vi "LV8_8.vi"() -> ()   [LabVIEW 2016]
uses:
  <vilib>/sound2/lvsound2.llb/Sampling Mode.ctl
  <vilib>/Utility/file.llb/Read From Spreadsheet File (DBL).vi
  <vilib>/imath/engines/lvmath2/RunTimeEngine/BuiltInFunctions/length/NIMS_length(GV).vi
  <instcachedir>/0/NIMS_length(GV)_08A3D13377FD4E4B96F5795FBF3698FA.lvgen/NIMS_length(GV)_08A3D13377FD4E4B96F5795FBF3698FA_000.vi
  <vilib>/imath/engines/lvmath2/RunTimeEngine/BuiltInFunctions/fft/NIMS_fft(GV).vi
  <instcachedir>/0/NIMS_fft(GV)_4C6467FC22F84E4BA42517A07EF978B0.lvgen/NIMS_fft(GV)_4C6467FC22F84E4BA42517A07EF978B0_000.vi
  <vilib>/imath/engines/lvmath2/RunTimeEngine/ErrorHandling/NIMS_Error From Error Code.vi
  <vilib>/imath/engines/lvmath2/RunTimeEngine/BuiltInFunctions/round/NIMS_round(DBL-S).vi
  <vilib>/imath/engines/lvmath2/RunTimeEngine/RangeToken/NIMS_Range_R2 - Integer.vi
  <instcachedir>/0/NIMS_Range_R2 - Integer_89B873E74E6E489885E44F751DD9C6BF.lvgen/NIMS_Range_R2 - Integer_89B873E74E6E489885E44F751DD9C6BF_000.vi
  <vilib>/imath/engines/lvmath2/RunTimeEngine/CommandStatement/MC_CommandStatement_break.vi
  <vilib>/imath/engines/lvmath2/RunTimeEngine/RowToken/NIMS_RowToken_M_SorRV.vi
  <instcachedir>/0/NIMS_RowToken_M_SorRV_4D710C5E6F8040F3A39B2F03436798DB.lvgen/NIMS_RowToken_M_SorRV_4D710C5E6F8040F3A39B2F03436798DB_000.vi
  <vilib>/imathl/engines/lvmath/Functions/Error Handling/Create Error.vi
  <vilib>/imath/engines/lvmath2/RunTimeEngine/RowToken/NIMS_RowToken_M_M.vi
  <instcachedir>/0/NIMS_RowToken_M_M_968CDE3545E74ACDAEA4B48DE01EEECA.lvgen/NIMS_RowToken_M_M_968CDE3545E74ACDAEA4B48DE01EEECA_004.vi
  <vilib>/imath/engines/lvmath2/RunTimeEngine/IndexReplace/NIMS V(M)=S.vi
  <instcachedir>/0/NIMS V(M)=S_9709F0D32A8A4ECDA1CDD54D8B4B61B5.lvgen/NIMS V(M)=S_9709F0D32A8A4ECDA1CDD54D8B4B61B5_000.vi
  <vilib>/imath/engines/lvmath2/RunTimeSupport/NIMS_Error if Not Equal.vi
  <instcachedir>/0/NIMS_Error if Not Equal_43252A79AD05436189442EC0C5E5AB8A.lvgen/NIMS_Error if Not Equal_43252A79AD05436189442EC0C5E5AB8A_002.vi
  <vilib>/imath/engines/lvmath2/RunTimeEngine/ErrorHandling/NIMS_Create Error From Enums.vi
  <vilib>/imath/engines/lvmath2/RunTimeEngine/BuiltInFunctions/ifft/NIMS_ifft(CV).vi
  <vilib>/imath/engines/lvmath2/RunTimeEngine/IndexRead/NIMS V(V).vi
  <instcachedir>/0/NIMS V(V)_298D9CB7BFEB42B8BC8D9C3C28AE8C70.lvgen/NIMS V(V)_298D9CB7BFEB42B8BC8D9C3C28AE8C70_000.vi
  <vilib>/imath/engines/lvmath2/RunTimeEngine/BuiltInFunctions/abs/NIMS_abs(signed).vi
  <instcachedir>/0/NIMS_abs(signed)_C4FCB8E6058B49B797C7C8D53CA5F6EC.lvgen/NIMS_abs(signed)_C4FCB8E6058B49B797C7C8D53CA5F6EC_006.vi
  <vilib>/imath/engines/lvmath2/RunTimeEngine/NodeEndStatement/NIMS_NodeEndStatement_Output.vi
  <instcachedir>/0/NIMS_NodeEndStatement_Output_53EC0D466D134D7ABD903AC30B43404B.lvgen/NIMS_NodeEndStatement_Output_53EC0D466D134D7ABD903AC30B43404B_005.vi
  <instcachedir>/0/NIMS_NodeEndStatement_Output_53EC0D466D134D7ABD903AC30B43404B.lvgen/NIMS_NodeEndStatement_Output_53EC0D466D134D7ABD903AC30B43404B_010.vi
  <vilib>/imath/engines/lvmath2/RunTimeEngine/ErrorHandling/NIMS_Finalize Error.vi
  <vilib>/sound2/lvsound2.llb/Sound Output Write (DBL Single).vi
panel:
  out "?":dbl
  in  "Fundamental rejection frequency":dbl(slide)=436.0 scale=400.0..500.0
  out "Filtered (frequency domain)":cluster{"F":dbl[], "FYI":dbl[]}(graph)
  out "Original signal (frequency domain)":cluster{"F":dbl[], "FXI":dbl[]}(graph)
  out "Original signal (time domain)":cluster{"t":dbl[], "first row":dbl[]}(graph)={"t"=[0.022675736961451247, 0.022698412698412697, 0.02272108843537415, 0.0227437641723356, 0.022766439909297054, 0.022789115646258504, 0.022811791383219954, 0.022834467120181407, 0.022857142857142857, 0.022879818594104307, 0.02290249433106576, 0.02292517006802721, 0.02294784580498866, 0.022970521541950114, 0.022993197278911564, 0.023015873015873017, 0.023038548752834467, 0.023061224489795917, 0.02308390022675737, 0.02310657596371882, 0.02312925170068027, 0.023151927437641724, 0.023174603174603174, 0.023197278911564624, 0.023219954648526078, 0.023242630385487528, 0.02326530612244898, 0.02328798185941043, 0.02331065759637188, 0.023333333333333334, 0.023356009070294784, 0.023378684807256234, 0.023401360544217688, 0.023424036281179138, 0.02344671201814059, 0.02346938775510204, 0.02349206349206349, 0.023514739229024945, 0.023537414965986395, 0.023560090702947845, 0.023582766439909298, 0.023605442176870748, 0.023628117913832198, 0.02365079365079365, 0.0236734693877551, 0.023696145124716555, 0.023718820861678005, 0.023741496598639455, 0.023764172335600908, 0.023786848072562358, 0.023809523809523808, 0.02383219954648526, 0.02385487528344671, 0.02387755102040816, 0.023900226757369615, 0.023922902494331065, 0.02394557823129252, 0.02396825396825397, 0.02399092970521542, 0.024013605442176872, 0.024036281179138322, 0.024058956916099772, 0.024081632653061225, 0.024104308390022675, 0.02412698412698413, 0.02414965986394558, 0.02417233560090703, 0.024195011337868482, 0.024217687074829932, 0.024240362811791382, 0.024263038548752835, 0.024285714285714285, 0.024308390022675735, 0.02433106575963719, 0.02435374149659864, 0.024376417233560092, 0.024399092970521542, 0.024421768707482992, 0.024444444444444446, 0.024467120181405896, 0.024489795918367346, 0.0245124716553288, 0.02453514739229025, 0.0245578231292517, 0.024580498866213153, 0.024603174603174603, 0.024625850340136056, 0.024648526077097506, 0.024671201814058956, 0.02469387755102041, 0.02471655328798186, 0.02473922902494331, 0.024761904761904763, 0.024784580498866213, 0.024807256235827663, 0.024829931972789116, 0.024852607709750566, 0.02487528344671202, 0.02489795918367347, 0.02492063492063492, 0.024943310657596373, 0.024965986394557823, 0.024988662131519273, 0.025011337868480726, 0.025034013605442176, 0.02505668934240363, 0.02507936507936508, 0.02510204081632653, 0.025124716553287983, 0.025147392290249433, 0.025170068027210883, 0.025192743764172337, 0.025215419501133787, 0.025238095238095237, 0.02526077097505669, 0.02528344671201814, 0.025306122448979593, 0.025328798185941043, 0.025351473922902493, 0.025374149659863947, 0.025396825396825397, 0.025419501133786847, 0.0254421768707483, 0.02546485260770975, 0.0254875283446712, 0.025510204081632654, 0.025532879818594104, 0.025555555555555557, 0.025578231292517007, 0.025600907029478457, 0.02562358276643991, 0.02564625850340136, 0.02566893424036281, 0.025691609977324264, 0.025714285714285714, 0.025736961451247164, 0.025759637188208617, 0.025782312925170067, 0.02580498866213152, 0.02582766439909297, 0.02585034013605442, 0.025873015873015874, 0.025895691609977324, 0.025918367346938774, 0.025941043083900227, 0.025963718820861677, 0.02598639455782313, 0.02600907029478458, 0.02603174603174603, 0.026054421768707484, 0.026077097505668934, 0.026099773242630384, 0.026122448979591838, 0.026145124716553288, 0.026167800453514738, 0.02619047619047619, 0.02621315192743764, 0.026235827664399095, 0.026258503401360545, 0.026281179138321994, 0.026303854875283448, 0.026326530612244898, 0.026349206349206348, 0.0263718820861678, 0.02639455782312925, 0.0264172335600907, 0.026439909297052155, 0.026462585034013605, 0.026485260770975058, 0.026507936507936508, 0.026530612244897958, 0.02655328798185941, 0.02657596371882086, 0.02659863945578231, 0.026621315192743765, 0.026643990929705215, 0.02666666666666667, 0.02668934240362812, 0.02671201814058957, 0.026734693877551022, 0.026757369614512472, 0.02678004535147392, 0.026802721088435375, 0.026825396825396825, 0.026848072562358275, 0.02687074829931973, 0.02689342403628118, 0.026916099773242632, 0.026938775510204082, 0.026961451247165532, 0.026984126984126985, 0.027006802721088435, 0.027029478458049885, 0.02705215419501134, 0.02707482993197279, 0.02709750566893424, 0.027120181405895692, 0.027142857142857142, 0.027165532879818596, 0.027188208616780046], "first row"=array[32768 elements]}
  out "Filtered signal (time domain)":cluster{"t":dbl[], "Y":dbl[]}(graph)={"t"=[0.022675736961451247, 0.022698412698412697, 0.02272108843537415, 0.0227437641723356, 0.022766439909297054, 0.022789115646258504, 0.022811791383219954, 0.022834467120181407, 0.022857142857142857, 0.022879818594104307, 0.02290249433106576, 0.02292517006802721, 0.02294784580498866, 0.022970521541950114, 0.022993197278911564, 0.023015873015873017, 0.023038548752834467, 0.023061224489795917, 0.02308390022675737, 0.02310657596371882, 0.02312925170068027, 0.023151927437641724, 0.023174603174603174, 0.023197278911564624, 0.023219954648526078, 0.023242630385487528, 0.02326530612244898, 0.02328798185941043, 0.02331065759637188, 0.023333333333333334, 0.023356009070294784, 0.023378684807256234, 0.023401360544217688, 0.023424036281179138, 0.02344671201814059, 0.02346938775510204, 0.02349206349206349, 0.023514739229024945, 0.023537414965986395, 0.023560090702947845, 0.023582766439909298, 0.023605442176870748, 0.023628117913832198, 0.02365079365079365, 0.0236734693877551, 0.023696145124716555, 0.023718820861678005, 0.023741496598639455, 0.023764172335600908, 0.023786848072562358, 0.023809523809523808, 0.02383219954648526, 0.02385487528344671, 0.02387755102040816, 0.023900226757369615, 0.023922902494331065, 0.02394557823129252, 0.02396825396825397, 0.02399092970521542, 0.024013605442176872, 0.024036281179138322, 0.024058956916099772, 0.024081632653061225, 0.024104308390022675, 0.02412698412698413, 0.02414965986394558, 0.02417233560090703, 0.024195011337868482, 0.024217687074829932, 0.024240362811791382, 0.024263038548752835, 0.024285714285714285, 0.024308390022675735, 0.02433106575963719, 0.02435374149659864, 0.024376417233560092, 0.024399092970521542, 0.024421768707482992, 0.024444444444444446, 0.024467120181405896, 0.024489795918367346, 0.0245124716553288, 0.02453514739229025, 0.0245578231292517, 0.024580498866213153, 0.024603174603174603, 0.024625850340136056, 0.024648526077097506, 0.024671201814058956, 0.02469387755102041, 0.02471655328798186, 0.02473922902494331, 0.024761904761904763, 0.024784580498866213, 0.024807256235827663, 0.024829931972789116, 0.024852607709750566, 0.02487528344671202, 0.02489795918367347, 0.02492063492063492, 0.024943310657596373, 0.024965986394557823, 0.024988662131519273, 0.025011337868480726, 0.025034013605442176, 0.02505668934240363, 0.02507936507936508, 0.02510204081632653, 0.025124716553287983, 0.025147392290249433, 0.025170068027210883, 0.025192743764172337, 0.025215419501133787, 0.025238095238095237, 0.02526077097505669, 0.02528344671201814, 0.025306122448979593, 0.025328798185941043, 0.025351473922902493, 0.025374149659863947, 0.025396825396825397, 0.025419501133786847, 0.0254421768707483, 0.02546485260770975, 0.0254875283446712, 0.025510204081632654, 0.025532879818594104, 0.025555555555555557, 0.025578231292517007, 0.025600907029478457, 0.02562358276643991, 0.02564625850340136, 0.02566893424036281, 0.025691609977324264, 0.025714285714285714, 0.025736961451247164, 0.025759637188208617, 0.025782312925170067, 0.02580498866213152, 0.02582766439909297, 0.02585034013605442, 0.025873015873015874, 0.025895691609977324, 0.025918367346938774, 0.025941043083900227, 0.025963718820861677, 0.02598639455782313, 0.02600907029478458, 0.02603174603174603, 0.026054421768707484, 0.026077097505668934, 0.026099773242630384, 0.026122448979591838, 0.026145124716553288, 0.026167800453514738, 0.02619047619047619, 0.02621315192743764, 0.026235827664399095, 0.026258503401360545, 0.026281179138321994, 0.026303854875283448, 0.026326530612244898, 0.026349206349206348, 0.0263718820861678, 0.02639455782312925, 0.0264172335600907, 0.026439909297052155, 0.026462585034013605, 0.026485260770975058, 0.026507936507936508, 0.026530612244897958, 0.02655328798185941, 0.02657596371882086, 0.02659863945578231, 0.026621315192743765, 0.026643990929705215, 0.02666666666666667, 0.02668934240362812, 0.02671201814058957, 0.026734693877551022, 0.026757369614512472, 0.02678004535147392, 0.026802721088435375, 0.026825396825396825, 0.026848072562358275, 0.02687074829931973, 0.02689342403628118, 0.026916099773242632, 0.026938775510204082, 0.026961451247165532, 0.026984126984126985, 0.027006802721088435, 0.027029478458049885, 0.02705215419501134, 0.02707482993197279, 0.02709750566893424, 0.027120181405895692, 0.027142857142857142, 0.027165532879818596, 0.027188208616780046], "Y"=array[32768 elements]}
  in  "Play original sound":bool
  in  "Play filtered sound":bool
  in  "stop":bool
  # "A note = 440 Hz"
  # "B note = 491 Hz"
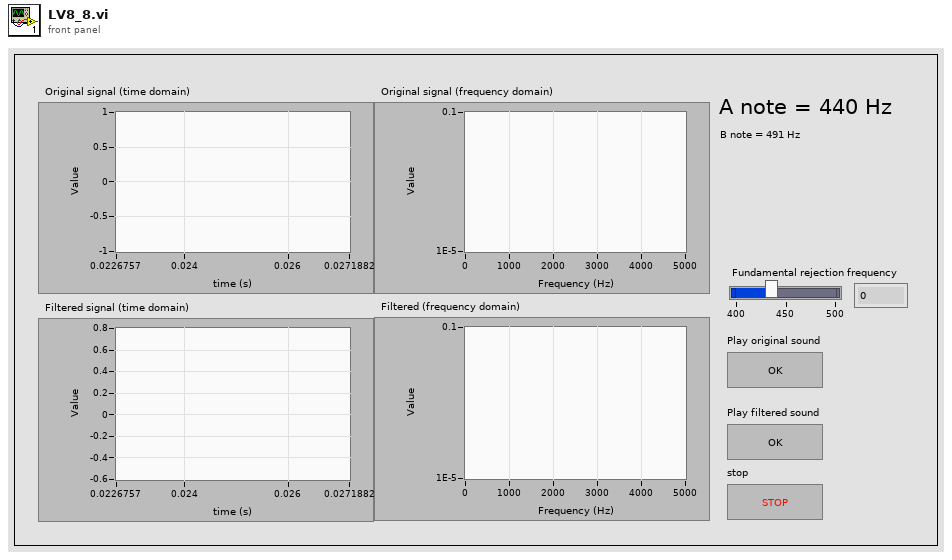
[diagram p1: front panel]
types:
  T1 = typedef "Sampling Mode.ctl" = i32
  T2 = typedef "Sound Output Task ID.ctl" = u32
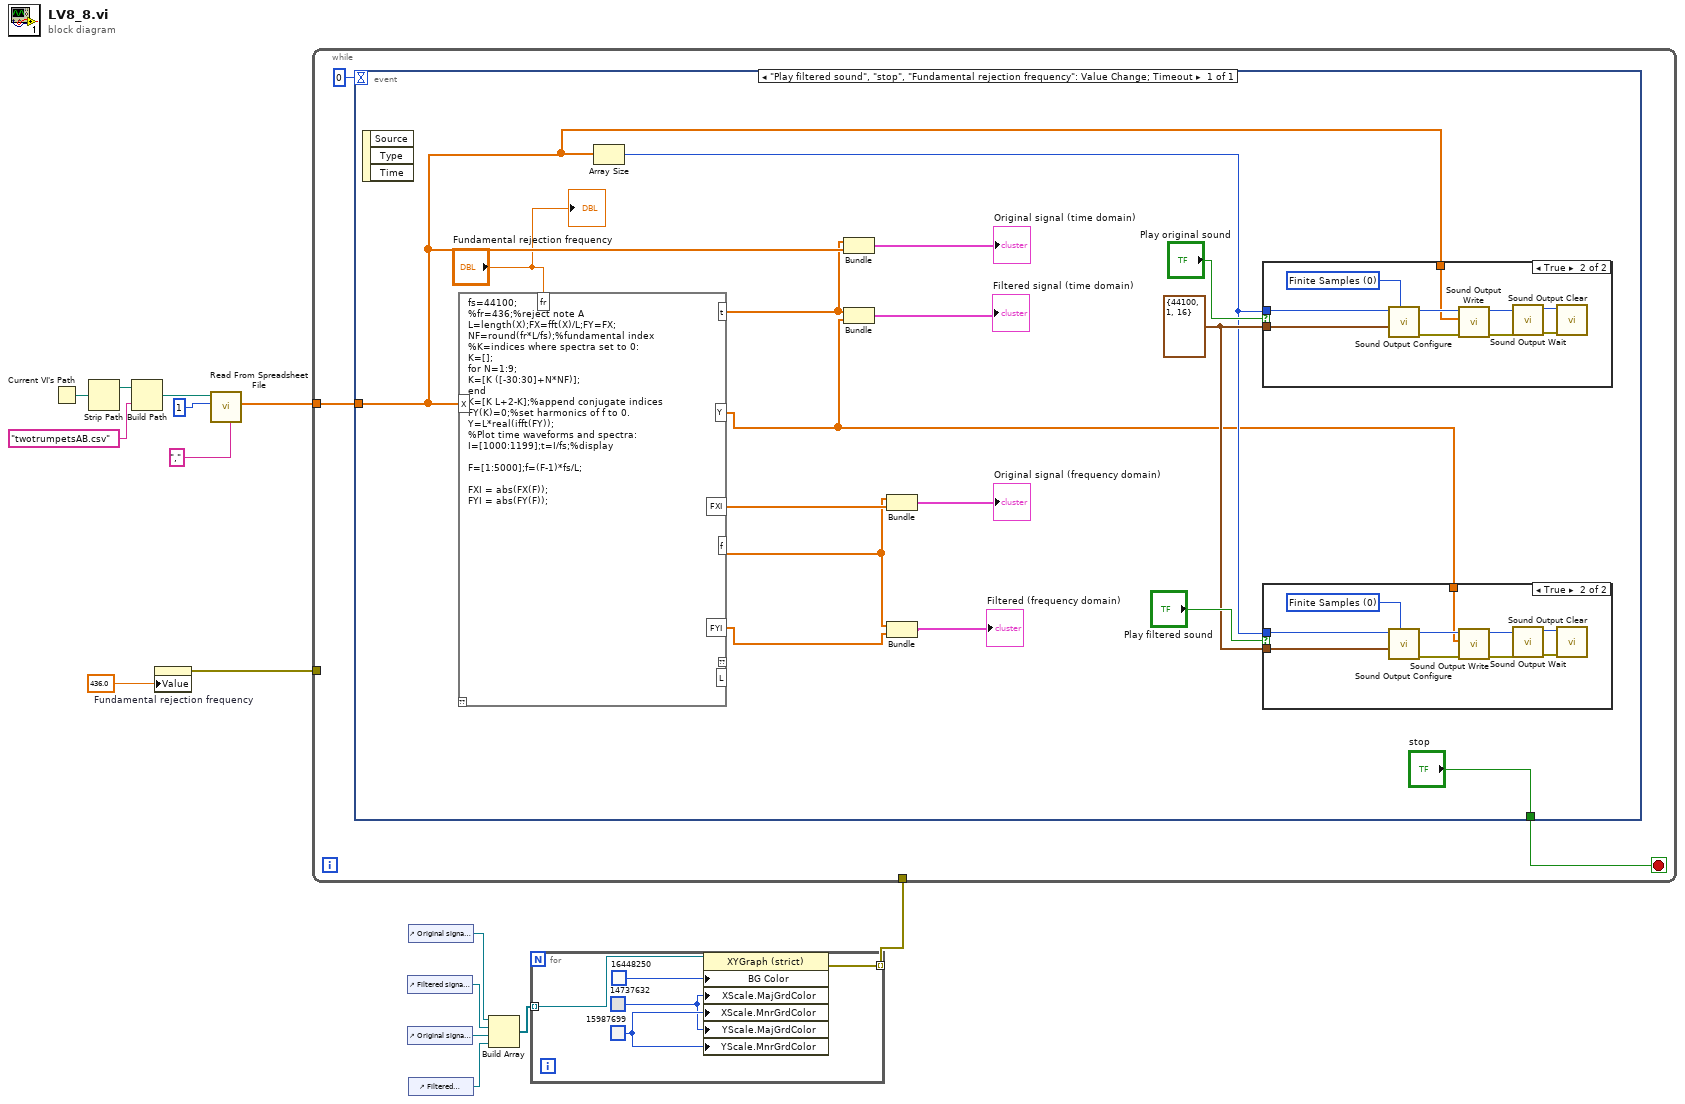
[diagram p0: block diagram]
diagram:
  n1 = Current VI's Path() -> (path=w15:path)
  n2 = Strip Path(path=w15) -> (stripped path=w14:path)  [unwired: 1 out]
  n3 = Build Path(base path=w14, name or relative path="twotrumpetsAB.csv") -> (appended path=w12:path)
  n4 = property on="Fundamental rejection frequency" class="Slide (strict)"("Value"=436.0 ("fundamental frequency")) -> (error out=w8:errorcluster)  [unwired: 2 in, 1 out]
  n5 = call-poly <vilib>:"Read From Spreadsheet File.vi"("delimiter (\\t)"="," ("delimiter (\\t)"), "number of rows (all:-1)"=1, "file path (dialog if empty)"=w12) -> ("first row"=w9:dbl[])  [unwired: 4 in, 4 out]
  n6 = control-ref of="Filtered signal (time domain)"() -> (w4:refnum<vi>)
  n7 = control-ref of="Original signal (frequency domain)"() -> (w3:refnum<vi>)
  n8 = control-ref of="Original signal (time domain)"() -> (w5:refnum<vi>)
  n9 = control-ref of="Filtered (frequency domain)"() -> (w2:refnum<vi>)
  n10 = Build Array(w5, w4, w3, w2) -> (w7:refnum<vi>[])
  n11 = for {
    tunnel: w7 -> [w17] mode=indexing
    tunnel: [w16] -> w6 mode=indexing
    w19 = u32 15987699
    w18 = u32 14737632
    n12 = property class="XYGraph (strict)"(reference=w17, "BG Color"=u32 16448250, "XScale.MajGrdColor"=w18, "XScale.MnrGrdColor"=w19, "YScale.MajGrdColor"=w18, "YScale.MnrGrdColor"=w19) -> (error out=w16:errorcluster)  [unwired: 1 in, 1 out]
  }
  n13 = while {
    tunnel: w9 -> [w23]
    tunnel: w8 -> [_]
    tunnel: w6 -> [_]
    stop <- w22 stop-if-true
    n14 = event shown="[0] \"Play filtered sound\", \"stop\", \"Fundamental rejection frequency\": Value Change;  Timeout" {
      selector: _ -> [_]
      dyn-events: _ -> [_]
      timeout: 0 -> [_]
      tunnel: w23 -> [w36]
      tunnel: ["stop"] -> w22
      event "Play filtered sound", "stop", "Fundamental rejection frequency": Value Change; Timeout {
        w34 = cluster{"fs":i32, i32, i32} {"fs"=44100, 1, 16}
        n15 = event-data() -> ()  [unwired: 1 in, 3 out]
        n16 = mathscript code="fs=44100;\n%fr=436;%reject note A\nL=length(X);FX=fft(X)/L;FY=FX;\nNF=round(fr*L/fs);%fundamental index\n%K=indices where spectra set to 0:\nK=[];\nfor N=1:9;\nK=[K ([-30:30]+N*NF)];\nend\nK=[K L+2-K];%append conjugate indices\nFY(K)=0;%set harmonics of f to 0.\nY=L*real(ifft(FY));\n%Plot time waveforms and spectra:\nI=[1000:1199];t=I/fs;%display\n\nF=[1:5000];f=(F-1)*fs/L;\n\nFXI = abs(FX(F));\nFYI = abs(FY(F));"("X"=w36, "fr"="Fundamental rejection frequency") -> ("Y"=w26:dbl[], "f"=w30:dbl[], "FYI"=w25:dbl[], "t"=w29:dbl[], "FXI"=w31:dbl[])  [unwired: 1 in, 2 out]
        n17 = Array Size(array=w36) -> (size(s)=w33:i32)
        n18 = Bundle("t"=w29, "first row"=w36) -> (→"Original signal (time domain)":cluster{"t":dbl[], "first row":dbl[]})  [unwired: 1 in]
        n19 = Bundle("t"=w29, "Y"=w26) -> (→"Filtered signal (time domain)":cluster{"t":dbl[], "Y":dbl[]})  [unwired: 1 in]
        n20 = Bundle("f"=w30, "FXI"=w31) -> (→"Original signal (frequency domain)":cluster{"f":dbl[], "FXI":dbl[]})  [unwired: 1 in]
        n21 = Bundle("f"=w30, "FYI"=w25) -> (→"Filtered (frequency domain)":cluster{"f":dbl[], "FYI":dbl[]})  [unwired: 1 in]
        n22 = case shown="True" "Play original sound" {
          tunnel: w34 -> [_ w325]
          tunnel: w33 -> [_ w323]
          tunnel: w36 -> [_ w322]
          frame False {
          }
          frame True {
            w324 = T1 0 items=["Finite Samples", "Continuous Samples"] ("sample mode")
            n23 = call <vilib>:"Sound Output Configure.vi"("number of samples/ch"=w323, "sample mode"=w324, "sound format"=w325) -> ("error out"=w326:errorcluster, "task ID"=w331:T2)  [unwired: 7 in]
            n24 = call-poly <vilib>:"Sound Output Write.vi"("error in (no error)"=w326, "data"=w322, "task ID"=w331) -> ("error out"=w327:errorcluster, "task ID out"=w328:T2)  [unwired: 7 in]
            n25 = call <vilib>:"Sound Output Wait.vi"("error in (no error)"=w327, "task ID"=w328) -> ("error out"=w330:errorcluster, "task ID out"=w329:T2)  [unwired: 8 in]
            n26 = call <vilib>:"Sound Output Clear.vi"("error in (no error)"=w330, "task ID"=w329) -> ()  [unwired: 9 in, 1 out]
          }
        }
        n27 = case shown="True" "Play filtered sound" {
          tunnel: w34 -> [_ w315]
          tunnel: w33 -> [_ w313]
          tunnel: w26 -> [_ w312]
          frame False {
          }
          frame True {
            w314 = T1 0 items=["Finite Samples", "Continuous Samples"] ("sample mode")
            n28 = call <vilib>:"Sound Output Configure.vi"("number of samples/ch"=w313, "sample mode"=w314, "sound format"=w315) -> ("error out"=w316:errorcluster, "task ID"=w321:T2)  [unwired: 7 in]
            n29 = call-poly <vilib>:"Sound Output Write.vi"("error in (no error)"=w316, "data"=w312, "task ID"=w321) -> ("error out"=w317:errorcluster, "task ID out"=w318:T2)  [unwired: 7 in]
            n30 = call <vilib>:"Sound Output Wait.vi"("error in (no error)"=w317, "task ID"=w318) -> ("error out"=w320:errorcluster, "task ID out"=w319:T2)  [unwired: 8 in]
            n31 = call <vilib>:"Sound Output Clear.vi"("error in (no error)"=w320, "task ID"=w319) -> ()  [unwired: 9 in, 1 out]
          }
        }
        "?" <- "Fundamental rejection frequency"
      }
    }
  }
